vi "LiveDataUpload.vi"(10 "Input Array":dbl[](array[numeric]), 11 "API String":string="V1WFARF28XTM5DW7") -> ()   [LabVIEW 2023]
uses:
  <vilib>/httpClient/LabVIEWHTTPClient.lvlib
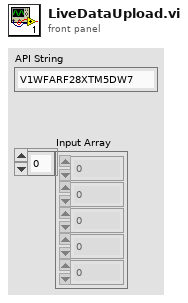
[diagram p1: front panel]
types:
  T1 = typedef "LabVIEWHTTPClient.lvlib/ClientHandle.ctl" = refnum<k1>
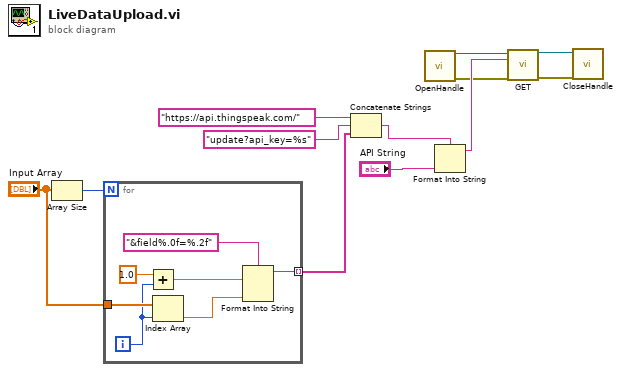
[diagram p0: block diagram]
diagram:
  n1 = Array Size(array="Input Array") -> (size(s)=w6:i32)
  n2 = for {
    N: w6 -> [_]
    tunnel: "Input Array" -> [w19]
    tunnel: [w16] -> w4 mode=indexing
    i -> [w13]
    n3 = Add(x=1.0, y=w13) -> (x+y=w15:dbl)
    n4 = Index Array(array=w19, index=w13) -> (element=w18:dbl)
    n5 = Format Into String(format string="&field%.0f=%.2f" ("string"), w15, w18) -> (resulting string=w16:string)  [unwired: 2 in, 1 out]
  }
  n6 = Concatenate Strings("https://api.thingspeak.com/" ("string"), "update?api_key=%s" ("string"), w4) -> (w7:string)
  n7 = call <vilib>:"OpenHandle.vi"() -> ("client handle out"=w11:T1, "error out"=w2:errorcluster)  [unwired: 14 in]
  n8 = Format Into String(format string=w7, "API String") -> (resulting string=w12:string)  [unwired: 2 in, 1 out]
  n9 = call <vilib>:"GET.vi"("client handle"=w11, "url"=w12, "error in (no error)"=w2) -> ("client handle out"=w9:T1, "error out"=w1:errorcluster)  [unwired: 9 in, 2 out]
  n10 = call <vilib>:"CloseHandle.vi"("client handle"=w9, "error in (no error)"=w1) -> ()  [unwired: 13 in, 1 out]
